vi "Build.vi"(8 "error in (no error)":errorcluster, 11 "Build in":refnum<class "AB_Build.lvclass">) -> (0 "error out":errorcluster, 1 "GeneratedFiles":path[](array[path]), 2 "GeneratedDirectories":path[](array[path]), 3 "Build out":refnum<class "AB_Build.lvclass">, 4 "GeneratedFileGUIDs":string[](array[string]), 5 "OutputDirectory":path, 7 "Dependencies":T1[](array[typedef]))   [LabVIEW 2020, in "AB_Build.lvclass"]
uses:
  <vilib>/AppBuilder/AB_Classes/Build/AB_Build.lvclass
  <vilib>/AppBuilder/AB_Dependency.ctl
  <vilib>/Utility/lvfile.llb/LVFileType.ctl
  <vilib>/AppBuilder/AB_Classes/Build/AB_Build.lvclass/AB_Build.ctl
  <vilib>/Utility/lvfile.llb/NI_FileType.lvlib
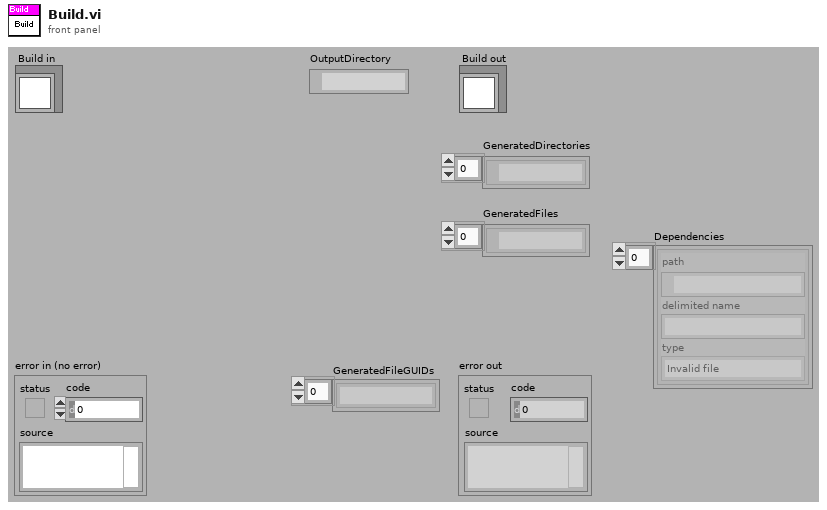
[diagram p1: front panel]
types:
  T1 = typedef "AB_Dependency.ctl" = cluster{"path":path, "delimited name":string, "type":T2}
  T2 = typedef "NI_FileType.lvlib/LVFileType.ctl" = enum32{"Invalid file", "Unknown type", "Instrument", "Control", "Polymorphic VI", "Project", "Library", "LVClass", "XControl", "XNode", "Shared library", ".NET assembly", "ActiveX interface", "CIN", "Run-time menu", "Palette menu", "Help file", "LLB", "XNode Edit Dependency", "Class Private Data Control", "Statechart", "MathScript .m file", "Ladder Diagram", "LVLibp", "XNode Build Dependency"}
  T3 = typedef "ItemRef.ctl" = u64
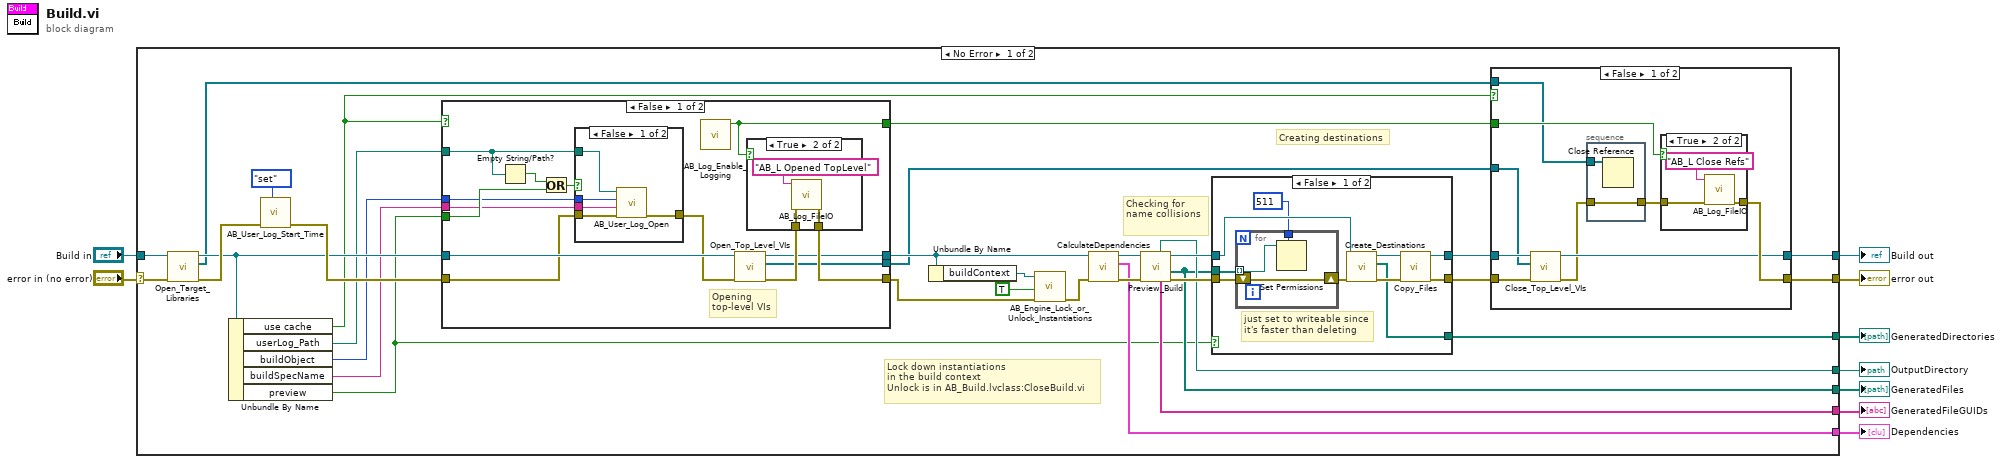
[diagram p0: block diagram]
diagram:
  n1 = case shown="No Error" "error in (no error)" {
    selector: "error in (no error)" -> [w20 w101]
    tunnel: [w26 w101] -> w2
    tunnel: [w24 w100] -> w7
    tunnel: "Build in" -> [w18 w100]
    tunnel: [w39 _] -> w6
    tunnel: [w33 _] -> w5
    tunnel: [w35 _] -> w4
    tunnel: [w34 _] -> w3
    tunnel: [w14 _] -> w1
    frame No Error {
      # "Lock down instantiations\nin the build context\nUnlock is in AB_Build.lvclass:CloseBuild.vi"
      # "Creating destinations"
      # "Checking for name collisions"
      n2 = call-dynamic "Open_Target_Libraries.vi"("error in (no error)"=w20, "Build in"=w18) -> ("error out"=w19:errorcluster, "Libraries"=w16:refnum<vi>[], "Build out"=w17:refnum<class "AB_Build.lvclass">)  [unwired: 7 in]
      n3 = Unbundle By Name(w17) -> ("use cache"=w15:bool, "userLog_Path"=w12:path, "buildObject"=w11:T3, "buildSpecName"=w10:string, "preview"=w13:bool)
      n4 = call <vilib>:"AB_User_Log_Start_Time.vi"("action"=enum16{"get", "set"}."set", "error in (no error)"=w19) -> ("error out"=w36:errorcluster)  [unwired: 9 out]
      n5 = case shown="False" w15 {
        tunnel: w36 -> [w48 w66]
        tunnel: [w55 _] -> w31
        tunnel: [w53 w66] -> w30
        tunnel: [w52 w67] -> w29
        tunnel: [w51 _] -> w23
        tunnel: w17 -> [w50 w67]
        tunnel: w13 -> [w46 _]
        tunnel: w12 -> [w44 _]
        tunnel: w11 -> [w43 _]
        tunnel: w10 -> [w42 _]
        frame False {
          # "Opening top-level VIs"
          n6 = Empty String/Path?(string/path=w44) -> (empty?=w45:bool)
          n7 = Or(x=w45, y=w46) -> (x .or. y?=w49:bool)
          n8 = case shown="False" w49 {
            tunnel: w48 -> [w60 w61]
            tunnel: [w56 w61] -> w47
            tunnel: w44 -> [w59 _]
            tunnel: w43 -> [w58 _]
            tunnel: w42 -> [w57 _]
            frame False {
              n9 = call <vilib>:"AB_User_Log_Open.vi"("error in (no error)"=w60, "build spec name"=w57, "Object"=w58, "file"=w59) -> ("error out"=w56:errorcluster)  [unwired: 7 out]
            }
            frame True {
            }
          }
          n10 = call <vilib>:"AB_Log_Enable_Logging.vi"() -> ("log?"=w55:bool)  [unwired: 2 in, 9 out]
          n11 = call-dynamic "Open_Top_Level_VIs.vi"("error in (no error)"=w47, "Build in"=w50) -> ("error out"=w54:errorcluster, "Top-Level VIs"=w51:refnum<vi>[], "Build out"=w52:refnum<class "AB_Build.lvclass">)  [unwired: 7 out]
          n12 = case shown="True" w55 {
            tunnel: w54 -> [w62 w64]
            tunnel: [w62 w63] -> w53
            frame False {
            }
            frame True {
              n13 = call <vilib>:"AB_Log_FileIO.vi"("error in (no error)"=w64, "newSection"="AB_L Opened TopLevel" ("sectionName")) -> ("error out"=w63:errorcluster)  [unwired: 3 in, 6 out]
            }
          }
        }
        frame True {
        }
      }
      n14 = Unbundle By Name(w29) -> ("buildContext"=w28:refnum<vi>)
      n15 = call <vilib>:"AB_Engine_Lock_or_Unlock_Instantiations.vi"("error in"=w30, "Lock?"=TRUE, "Instance to Lock or Unlock"=w28) -> ("error out"=w21:errorcluster)  [unwired: 8 in]
      n16 = call-dynamic "CalculateDependencies.vi"("error in (no error)"=w21, "Build in"=w29) -> ("error out"=w37:errorcluster, "Dependencies"=w14:T1[], "Build out"=w38:refnum<class "AB_Build.lvclass">)  [unwired: 1 in, 6 out]
      n17 = call-dynamic "Preview_Build.vi"("error in (no error)"=w37, "Build in"=w38) -> ("error out"=w40:errorcluster, "GeneratedFiles"=w33:path[], "Build out"=w41:refnum<class "AB_Build.lvclass">, "GeneratedFileGUIDs"=w35:string[], "OutputDirectory"=w34:path)  [unwired: 5 out]
      n18 = case shown="False" w13 {
        tunnel: w41 -> [w87 w98]
        tunnel: [w94 w98] -> w25
        tunnel: w40 -> [w89 w99]
        tunnel: [w93 w99] -> w22
        tunnel: [w90 _] -> w39
        tunnel: w33 -> [w86 _]
        frame False {
          # "just set to writeable since\nit's faster than deleting"
          n19 = for {
            shift-right: [w97] -> w88
            shift-left: w89 -> [w97]
            tunnel: w86 -> [w96] mode=indexing
            tunnel: i16 511 ("permissions") -> [w95]
            n20 = Set Permissions(7:w95, 11:w96) -> ()  [unwired: 1 in, 4 out]
          }
          n21 = call-dynamic "Create_Destinations.vi"("error in (no error)"=w88, "Build in"=w87) -> ("error out"=w91:errorcluster, "createdDirectories"=w90:path[], "Build out"=w92:refnum<class "AB_Build.lvclass">)  [unwired: 7 out]
          n22 = call-dynamic "Copy_Files.vi"("error in (no error)"=w91, "Build in"=w92) -> ("error out"=w93:errorcluster, "Build out"=w94:refnum<class "AB_Build.lvclass">)  [unwired: 8 out]
        }
        frame True {
        }
      }
      n23 = case shown="False" w15 {
        tunnel: w31 -> [w76 _]
        tunnel: [w75 w83] -> w26
        tunnel: w25 -> [w74 w84]
        tunnel: [w73 w84] -> w24
        tunnel: w23 -> [w72 _]
        tunnel: w22 -> [w71 w83]
        tunnel: w16 -> [w68 _]
        frame False {
          n24 = call-dynamic "Close_Top_Level_VIs.vi"("error in (no error)"=w71, "Top-Level VIs"=w72, "AB_Build in"=w74) -> ("error out"=w70:errorcluster, "AB_Build out"=w73:refnum<class "AB_Build.lvclass">)  [unwired: 7 in]
          n25 = stacked-sequence {
            tunnel: [w78] -> w69
            tunnel: w70 -> [w78]
            tunnel: w68 -> [w77]
            frame #0 {
              n26 = Close Reference(reference=w77) -> ()  [unwired: 1 in, 1 out]
            }
          }
          n27 = case shown="True" w76 {
            tunnel: w69 -> [w79 w82]
            tunnel: [w79 w81] -> w75
            frame False {
            }
            frame True {
              n28 = call <vilib>:"AB_Log_FileIO.vi"("error in (no error)"=w82, "newSection"="AB_L Close Refs" ("sectionName")) -> ("error out"=w81:errorcluster)  [unwired: 3 in, 6 out]
            }
          }
        }
        frame True {
        }
      }
    }
    frame Error {
    }
  }
  "error out" <- w2
  "Build out" <- w7
  "GeneratedDirectories" <- w6
  "GeneratedFiles" <- w5
  "GeneratedFileGUIDs" <- w4
  "OutputDirectory" <- w3
  "Dependencies" <- w1
